vi "Change Receive Window Size.vi"(8 "Error In":errorcluster, 9 "Force":u8, 10 "Size":u32, 11 "Channel In":refnum<class "Channel.lvclass">) -> (0 "Error Out":errorcluster, 2 "Window":u32, 3 "Channel Out":refnum<class "Channel.lvclass">)   [LabVIEW 2018, in "Toolkit.lvlib" / "Channel.lvclass"]
doc: "Adjusts the receive window size in bytes."
uses:
  Channel.lvclass
  Channel.lvclass/Channel.ctl
  Session/Session.lvclass/Session.ctl
  SSH/SSH.lvclass/SSH.ctl
  Session/Session.lvclass
  Toolkit.lvlib
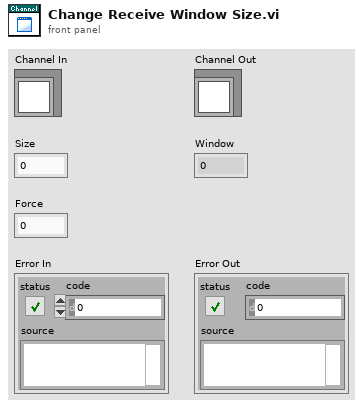
[diagram p1: front panel]
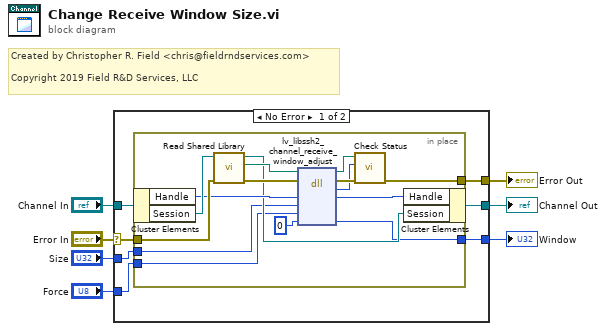
[diagram p0: block diagram]
diagram:
  # "Created by Christopher R. Field <chris@fieldrndservices.com>\n\nCopyright 2019 Field R&D Services, LLC"
  n1 = case shown="No Error" "Error In" {
    selector: "Error In" -> [w12 w31]
    tunnel: [w11 w31] -> w6
    tunnel: "Channel In" -> [w14 w30]
    tunnel: [w13 w30] -> w4
    tunnel: "Size" -> [w10 _]
    tunnel: "Force" -> [w9 _]
    tunnel: [w8 _] -> w1
    frame No Error {
      n2 = in-place {
        in-place-border: w12 -> [w26]
        in-place-border: [w22] -> w11
        in-place-border: w10 -> [w18]
        in-place-border: w9 -> [w17]
        in-place-border: [w15] -> w8
        n3 = in-place-cluster #1(w14) -> ("Handle"=w21:u64, "Session"=w29:refnum<class "Session.lvclass">)
        n4 = call "Read Shared Library.vi"("Error In"=w26, "Session In"=w29) -> ("Erorr Out"=w27:errorcluster, "libssh2lv Shared Library"=w28:path, "Session Out"=w19:refnum<class "Session.lvclass">)  [unwired: 7 in]
        n5 = dll-call lib="libssh2lv.*" fn="lv_libssh2_channel_receive_window_adjust"(path in=w28, error in=w27, "handle"=w21, "adjustment"=w18, "force"=w17, "window"=u32 0) -> (path out=w24:path, error out=w25:errorcluster, "status"=w23:i32, "handle"=w20:u64, "window"=w15:u32)  [unwired: 3 in]
        n6 = call "Check Status.vi"("Error In"=w25, "Status"=w23, "lv-libssh2 Shared Library In"=w24) -> ("Error Out"=w22:errorcluster)  [unwired: 7 in, 1 out]
        n7 = in-place-cluster #1("Handle"=w20, "Session"=w19) -> (w13:refnum<class "Channel.lvclass">)
      }
    }
    frame Error {
    }
  }
  "Error Out" <- w6
  "Channel Out" <- w4
  "Window" <- w1
